vi "Coerce_and_Center_Coords.vi"(0 "Coords_In":T1, 1 "Feature_Size":i32) -> (5 "Coords_Out":T1)   [LabVIEW 2020]
uses:
  Controls/Dims(2D)ctl.ctl
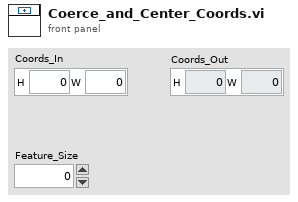
[diagram p1: front panel]
types:
  T1 = typedef "Dims(2D)ctl.ctl" = cluster{"H":i32, "W":i32}
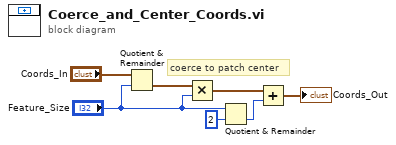
[diagram p0: block diagram]
diagram:
  # "coerce to patch center"
  n1 = Quotient & Remainder(x="Coords_In", y="Feature_Size") -> (floor(x/y)=w2:T1)  [unwired: 1 out]
  n2 = Multiply(x=w2, y="Feature_Size") -> (x*y=w3:T1)
  n3 = Quotient & Remainder(x="Feature_Size", y=2) -> (floor(x/y)=w4:i32)  [unwired: 1 out]
  n4 = Add(x=w3, y=w4) -> (x+y=→"Coords_Out":T1)
